vi "ODC.vi"(0 "System no.":i32=1 min=1 max=4 step=1, 2 "Axes to set":string[](array[string]), 3 "Deceleration values":dbl[](array[numeric]) format="%.6f", 4 "No.of digits":i16=4, 5 "error in":errorcluster, 6 "Without axis ID?":bool) -> (14 "Controller error":bool, 19 "error out":errorcluster)   [LabVIEW 2020]
doc: "Sets open-loop deceleration and checks for error. If Without axis ID? is TRUE, then Axes to set is ignored and first field of Deceleration values array is used for deceleration command. Number of digits is the number of digits after the decimal point in the deceleration value(s) that will be sent. Controller error is TRUE if selected system reports error code which is not 0.\n\nE-861, E-874: Without axis ID? = FALSE. Deceleration unit is steps/s²."
panel:
  # "Sets open-loop deceleration and checks for error.  If \"Without\naxis ID\" is TRUE, then \"Axes to set\" is ignored and first field of \nDeceleration values\" array is used for deceleration command."
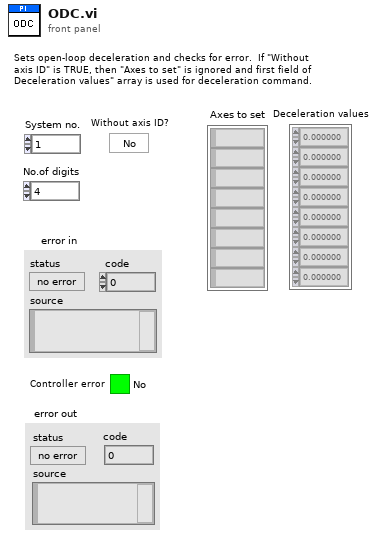
[diagram p1: front panel]
types:
  T1 = enum16{"Disable error check", "Force error check", "Use global settings"}
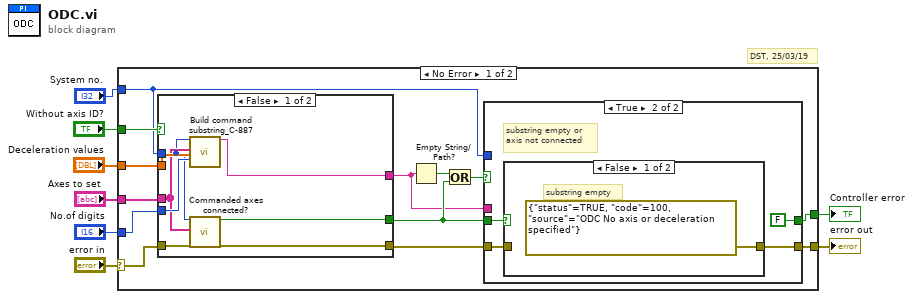
[diagram p0: block diagram]
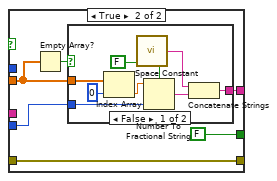
[diagram p2: hidden frame]
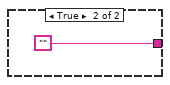
[diagram p3: hidden frame]
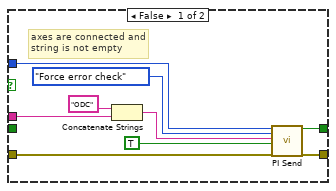
[diagram p4: hidden frame]
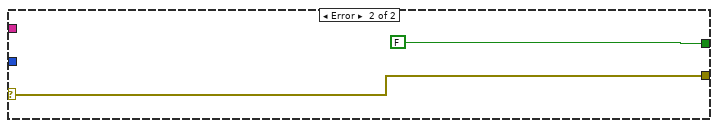
[diagram p6: hidden frame]
diagram:
  # "DST, 25/03/19"
  n1 = case shown="No Error" "error in" {
    selector: "error in" -> [w10 w61]
    tunnel: [w21 w61] -> w8
    tunnel: "Deceleration values" -> [w20 _]
    tunnel: "No.of digits" -> [w19 _]
    tunnel: "System no." -> [w14 _]
    tunnel: "Axes to set" -> [w17 _]
    tunnel: "Without axis ID?" -> [w15 _]
    tunnel: [w9 FALSE ("Controller error")] -> w1
    frame No Error {
      n2 = case shown="False" w15 {
        tunnel: [w29 w33] -> w11
        tunnel: w20 -> [w28 w31]
        tunnel: w19 -> [w27 w32]
        tunnel: w10 -> [w26 w35]
        tunnel: [w25 w35] -> w18
        tunnel: w14 -> [w22 _]
        tunnel: w17 -> [w24 _]
        tunnel: [w23 FALSE] -> w13
        frame False {
          n3 = call "Build command substring_C-887.vi"("System no."=w22, "Affected axes"=w24, "Parameters"=w28, "No. of digits"=w27) -> ("Command substring"=w29:string)  [unwired: 3 in, 12 out]
          n4 = call "Commanded axes connected?.vi"("System no."=w22, "Commanded axes"=w24, "error in"=w26) -> ("Controller error"=w23:bool, "error out"=w25:errorcluster)  [unwired: 1 in, 14 out]
        }
        frame True {
          n5 = Empty Array?(array=w31) -> (empty?=w30:bool)
          n6 = case shown="False" w30 {
            tunnel: [w41 ""] -> w33
            tunnel: w31 -> [w40 _]
            tunnel: w32 -> [w38 _]
            frame False {
              n7 = Index Array(array=w40, index=0 ("Index")) -> (element=w39:dbl)
              n8 = call <vilib>:"Space Constant.vi"() -> ("String"=w42:string)
              n9 = Number To Fractional String(use system decimal point (T)=FALSE, number=w39, precision (6)=w38) -> (F-format string=w37:string)  [unwired: 1 out]
              n10 = Concatenate Strings(w42, w37) -> (w41:string)
            }
            frame True {
            }
          }
        }
      }
      n11 = Empty String/Path?(string/path=w11) -> (empty?=w12:bool)
      n12 = Or(x=w12, y=w13) -> (x .or. y?=w16:bool)
      n13 = case shown="True" w16 {
        tunnel: w11 -> [w52 _]
        tunnel: [w46 w57] -> w21
        tunnel: w18 -> [w49 w55]
        tunnel: w13 -> [_ w56]
        tunnel: w14 -> [w48 _]
        tunnel: [w45 FALSE ("Controller error")] -> w9
        frame False {
          # "axes are connected and\nstring is not empty"
          n14 = Concatenate Strings("ODC", w52) -> (w50:string)
          n15 = call "PI Send.vi"("System no."=w48, "Error check settings"=T1."Force error check", "String to send"=w50, "Attach termination char.?"=TRUE ("Attach Linefeed?"), "error in"=w49) -> ("Controller error"=w45:bool, "error out"=w46:errorcluster)  [unwired: 1 in, 12 out]
        }
        frame True {
          # "substring empty or\naxis not connected"
          n16 = case shown="False" w56 {
            tunnel: [errorcluster {"status"=TRUE, "code"=100, "source"="ODC No axis or deceleration specified"} ("error out") w59] -> w57
            tunnel: w55 -> [_ w59]
            frame False {
              # "substring empty"
            }
            frame True {
              # "commanded axis\nnot connected"
            }
          }
        }
      }
    }
    frame Error {
    }
  }
  "error out" <- w8
  "Controller error" <- w1
